vi "UpdateMachineGaps.vi"(8 "u( Machine Index)":i32, 9 "Operation Finish Time":i32, 10 "Operation Start Time":i32, 11 "Machine Gaps in":T1[][](array[typedef])) -> (3 "Machine Gaps out":T1[][](array[typedef]))   [LabVIEW 2013, in "Scheduler.lvclass"]
uses:
  Scheduler.lvclass
  Controls/GapStructure4FIFOEngine.ctl
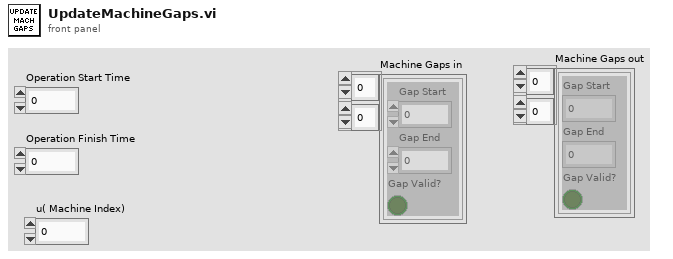
[diagram p1: front panel]
types:
  T1 = typedef "Scheduler.lvclass/GapStructure4FIFOEngine.ctl" = cluster{"Gap Start":i32, "Gap End":i32, "Gap Valid?":bool}
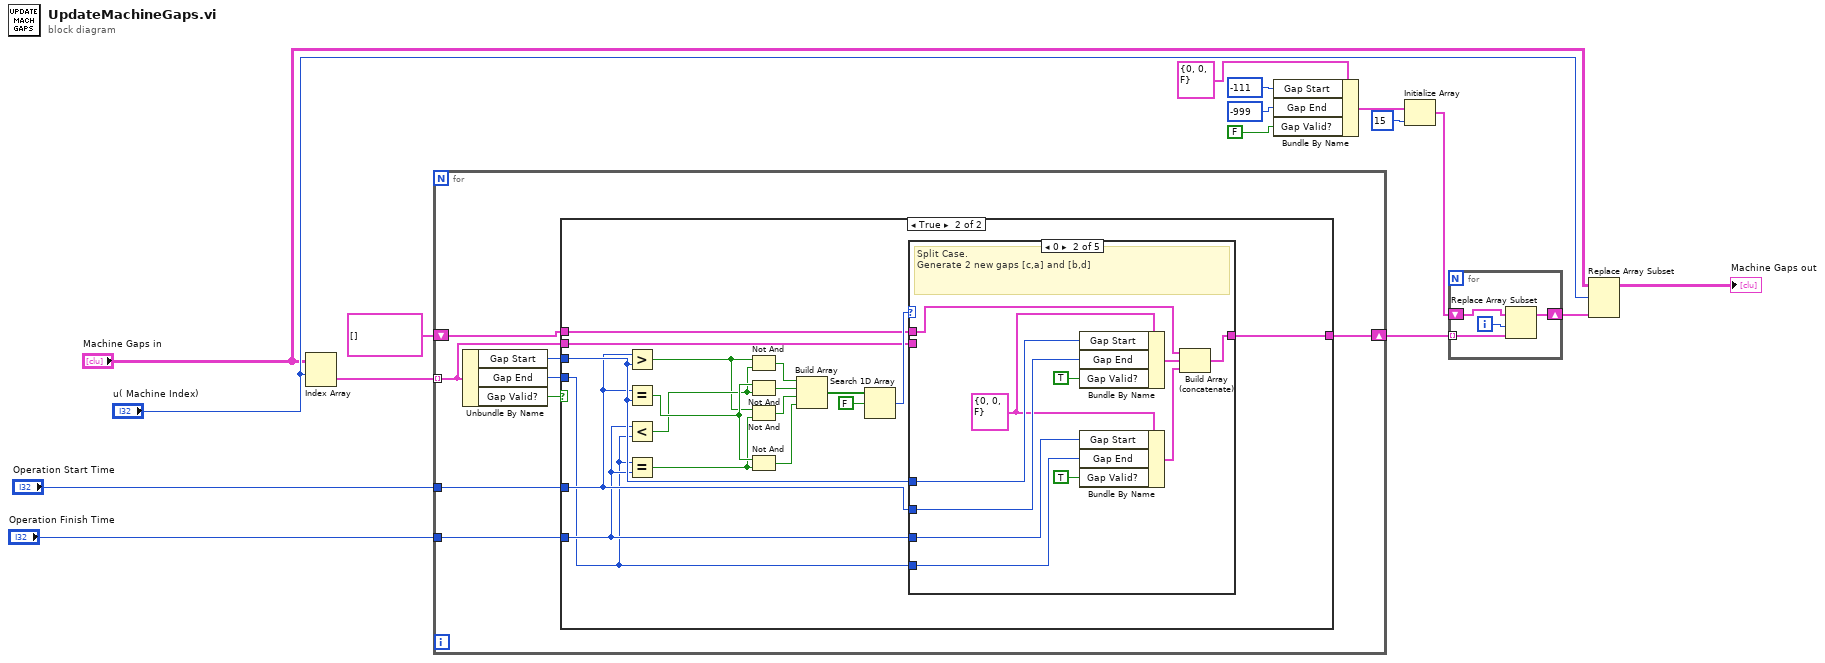
[diagram p0: block diagram]
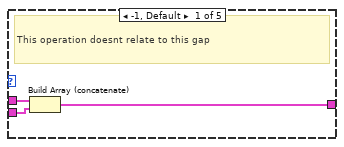
[diagram p3: hidden frame]
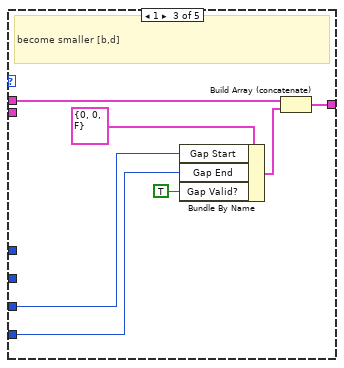
[diagram p4: hidden frame]
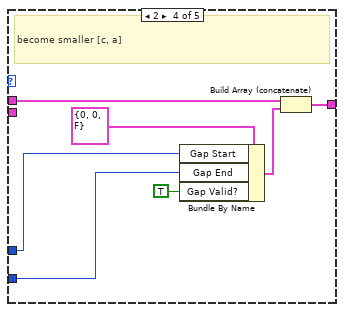
[diagram p5: hidden frame]
diagram:
  n1 = Index Array(array="Machine Gaps in", index (row)="u( Machine Index)") -> (element=w11:T1[])  [unwired: 1 in]
  n2 = for {
    tunnel: w11 -> [w17] mode=indexing
    tunnel: "Operation Finish Time" -> [w23]
    tunnel: "Operation Start Time" -> [w22]
    shift-right: [w18] -> w9
    shift-left: T1[] [] -> [w19]
    n3 = Unbundle By Name(w17) -> ("Gap Start"=w21:i32, "Gap End"=w20:i32, "Gap Valid?"=w24:bool)
    n4 = case shown="True" w24 {
      tunnel: w23 -> [_ w28]
      tunnel: w22 -> [_ w29]
      tunnel: w21 -> [_ w30]
      tunnel: w20 -> [_ w27]
      tunnel: w19 -> [w25 w32]
      tunnel: [w25 w31] -> w18
      tunnel: w17 -> [_ w26]
      frame False {
      }
      frame True {
        n5 = Greater?(x=w29, y=w30) -> (0:w38:bool)
        n6 = Equal?(x=w29, y=w30) -> (x = y?=w41:bool)
        n7 = Less?(x=w28, y=w27) -> (x < y?=w40:bool)
        n8 = Equal?(x=w27, y=w28) -> (x = y?=w37:bool)
        n9 = Not And(1:w40, 2:w38) -> (0:w42:bool)
        n10 = Not And(1:w40, 2:w41) -> (0:w39:bool)
        n11 = Not And(1:w37, 2:w38) -> (0:w36:bool)
        n12 = Not And(1:w37, 2:w41) -> (0:w43:bool)
        n13 = Build Array(w42, w39, w36, w43) -> (w35:bool[])
        n14 = Search 1D Array(1D array=w35, element=FALSE) -> (index of element=w33:i32)  [unwired: 1 in]
        n15 = case shown="0" w33 {
          tunnel: w32 -> [w45 w48 w59 w69 w72]
          tunnel: [w44 w47 w58 w68 w72] -> w31
          tunnel: w30 -> [_ w56 _ w66 _]
          tunnel: w29 -> [_ w55 _ w65 _]
          tunnel: w28 -> [_ w52 w63 _ _]
          tunnel: w27 -> [_ w51 w62 _ _]
          tunnel: w26 -> [w46 _ _ _ _]
          frame -1, Default {
            # "This operation doesnt relate to this gap"
            n16 = Build Array (concatenate)(w45, w46) -> (w44:T1[])
          }
          frame 0 {
            w53 = T1 {"Gap Start"=0, "Gap End"=0, "Gap Valid?"=FALSE}
            # "Split Case.\nGenerate 2 new gaps [c,a] and [b,d]"
            n17 = Bundle By Name(cluster=w53, "Gap Start"=w56, "Gap End"=w55, "Gap Valid?"=TRUE) -> (w54:T1)
            n18 = Bundle By Name(cluster=w53, "Gap Start"=w52, "Gap End"=w51, "Gap Valid?"=TRUE) -> (w49:T1)
            n19 = Build Array (concatenate)(w48, w54, w49) -> (w47:T1[])
          }
          frame 1 {
            # "become smaller [b,d]"
            n20 = Bundle By Name(cluster=T1 {"Gap Start"=0, "Gap End"=0, "Gap Valid?"=FALSE}, "Gap Start"=w63, "Gap End"=w62, "Gap Valid?"=TRUE) -> (w60:T1)
            n21 = Build Array (concatenate)(w59, w60) -> (w58:T1[])
          }
          frame 2 {
            # "become smaller [c, a]"
            n22 = Bundle By Name(cluster=T1 {"Gap Start"=0, "Gap End"=0, "Gap Valid?"=FALSE}, "Gap Start"=w66, "Gap End"=w65, "Gap Valid?"=TRUE) -> (w70:T1)
            n23 = Build Array (concatenate)(w69, w70) -> (w68:T1[])
          }
          frame 3 {
            # "gap disappears"
          }
        }
      }
    }
  }
  n24 = Bundle By Name(cluster=T1 {"Gap Start"=0, "Gap End"=0, "Gap Valid?"=FALSE}, "Gap Start"=-111, "Gap End"=-999, "Gap Valid?"=FALSE) -> (w4:T1)
  n25 = Initialize Array(w4, 15 ("dimension size")) -> (w2:T1[])
  n26 = for {
    tunnel: w9 -> [w74] mode=indexing
    shift-right: [w73] -> w1
    shift-left: w2 -> [w76]
    i -> [w75]
    n27 = Replace Array Subset(array=w76, new element=w74, index=w75) -> (w73:T1[])
  }
  n28 = Replace Array Subset(array="Machine Gaps in", new element=w1, index (row)="u( Machine Index)") -> (→"Machine Gaps out":T1[][])  [unwired: 1 in]
